vi "py_control_test.vi"() -> ()   [LabVIEW 2025]
panel:
  in  "Cluster":T1
  in  "PIDGains":T2={"proportional gain (Kc)"=1.0, "integral time (Ti, min)"=0.01, "derivative time (Td, min)"=0.0} {"derivative time (Td, min)" format="%.3f"; "integral time (Ti, min)" format="%.3f"; "proportional gain (Kc)" format="%.3f"}
  in  "StringControl":string
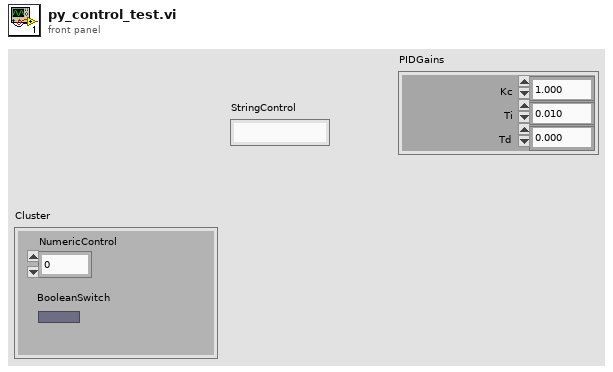
[diagram p1: front panel]
types:
  T1 = cluster{"NumericControl":dbl, "BooleanSwitch":bool}
  T2 = cluster{"proportional gain (Kc)":dbl, "integral time (Ti, min)":dbl, "derivative time (Td, min)":dbl}
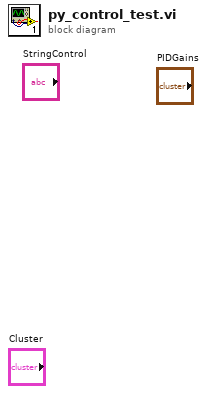
[diagram p0: block diagram]
diagram:
